vi "_Obtain JKISMQ.vi"(8 "Error in":errorcluster caption="Error in (no error)", 9 "create if not found? (T)":bool=TRUE, 11 "Name(\"\" to use uuid) in":string) -> (0 "Error out":errorcluster, 3 "JKISMQ":T1, 4 "Name":string)   [LabVIEW 2014, in "JKI-State-Machine-Plus.lvlib"]
uses:
  JKI-State-Machine-Plus.lvlib
  _JKISMQ.ctl
  Typedef/_Cross JKI StateMachine State Data.ctl
  Typedef/_JKISM_MSG_TYPE.ctl
  Typedef/_Cross JKI StateMachine State Response.ctl
  Typedef/_JKISM_MODE.ctl
  _JKISMQFGVOPER.ctl
  FGV-BroadcastRegistry/global-JKISMQFGVChangeTStamp.vi
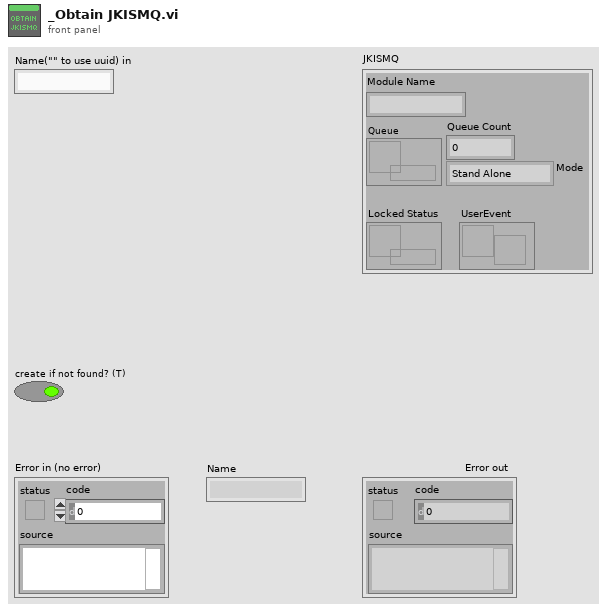
[diagram p1: front panel]
types:
  T1 = typedef "JKI-State-Machine-Plus.lvlib/_JKISMQ.ctl" = cluster{"Module Name":string, "Queue":refnum<queue>, "Locked Status":refnum<data-value>, "Mode":T2, "UserEvent":refnum<user-event>, "Queue Count":i32}
  T2 = typedef "JKI-State-Machine-Plus.lvlib/_JKISM_MODE.ctl" = enum16{"Stand Alone", "JKISM", "Dispatch Worker"}
  T3 = typedef "JKI-State-Machine-Plus.lvlib/_JKISMQFGVOPER.ctl" = enum16{"Get By Name", "List", "Check If Name Exists", "Release", "Module Status"}
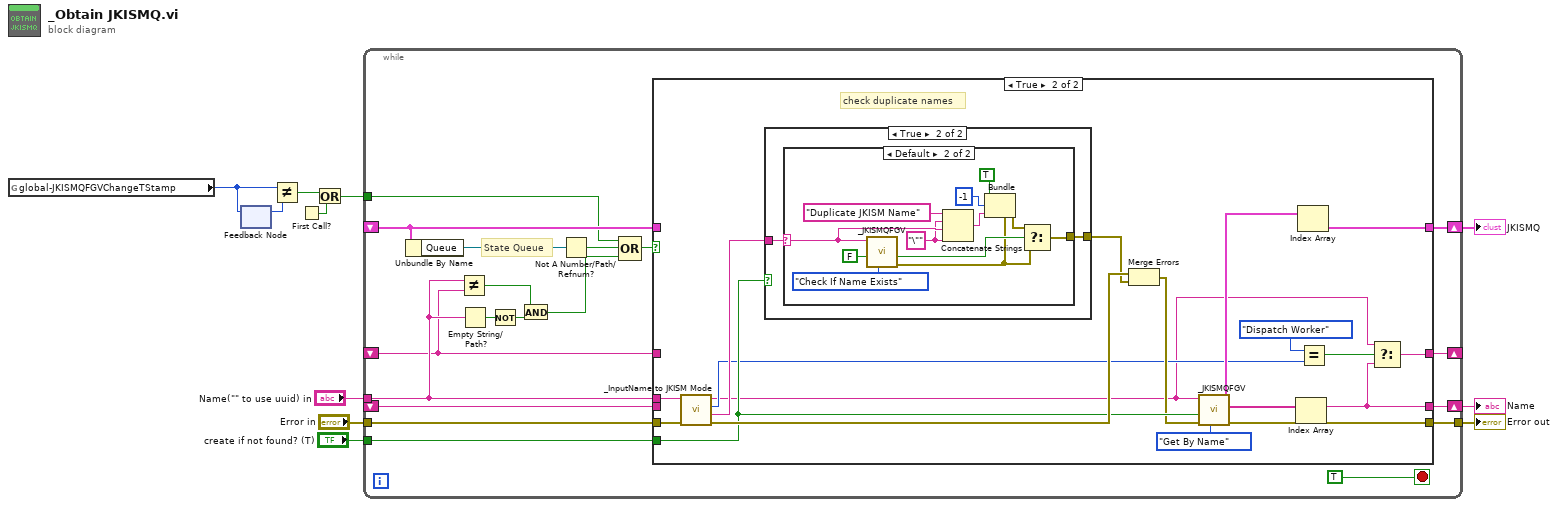
[diagram p0: block diagram]
diagram:
  n1 = global read "global-JKISMQFGVChangeTStamp.vi" "global-JKISMQFGVChangeTStamp"() -> (w2:u32)
  n2 = feedback #1() -> (w3:u32)  [unwired: 1 in]
  n3 = feedback-in #1(w2) -> ()
  n4 = Not Equal?(x=w2, y=w3) -> (x != y?=w5:bool)
  n5 = First Call?() -> (First Call?: T/F=w4:bool)
  n6 = Or(x=w5, y=w4) -> (x .or. y?=w1:bool)
  n7 = while {
    shift-right: [w28] -> w11
    shift-left: _ -> [w23]
    shift-right: [w27] -> w6
    shift-left: _ -> [w19]
    tunnel: "create if not found? (T)" -> [w26]
    tunnel: "Error in" -> [w25]
    tunnel: [w24] -> w8
    tunnel: "Name(\"\" to use uuid) in" -> [w20]
    shift-right: [w14] -> _
    shift-left: _ -> [w13]
    tunnel: w1 -> [w12]
    stop <- TRUE stop-if-true
    # "State Queue"
    n8 = Unbundle By Name(w19) -> ("Queue"=w18:refnum<queue>)
    n9 = Not Equal?(x=w20, y=w13) -> (x != y?=w17:bool)
    n10 = Empty String/Path?(string/path=w20) -> (empty?=w16:bool)
    n11 = Not(x=w16) -> (.not. x?=w15:bool)
    n12 = And(x=w17, y=w15) -> (x .and. y?=w21:bool)
    n13 = Not A Number/Path/Refnum?(number/path/refnum=w18) -> (NaN/Path/Refnum?=w29:bool)
    n14 = Compound Arithmetic op=OR(w12, w29, w21) -> (w22:bool)
    n15 = case shown="True" w22 {
      tunnel: w23 -> [w34 _]
      tunnel: [w34 w36] -> w28
      tunnel: [w33 w43] -> w27
      tunnel: w19 -> [w33 _]
      tunnel: w26 -> [_ w46]
      tunnel: w25 -> [w32 w48]
      tunnel: [w32 w47] -> w24
      tunnel: w20 -> [_ w42]
      tunnel: [w31 w35] -> w14
      tunnel: w13 -> [w31 _]
      frame False {
      }
      frame True {
        # "check duplicate names"
        n16 = call "_InputName to JKISM Mode.vi"("String"=w42) -> ("QName"=w41:string, "JKISM Mode"=w40:T2, "String(dup)"=w37:string)  [unwired: 8 in]
        n17 = case shown="True" w46 {
          tunnel: w41 -> [_ w52]
          tunnel: [_ w53] -> w44
          frame False {
          }
          frame True {
            n18 = case shown="Default" w52 {
              selector: w52 -> [_ w56]
              tunnel: [_ w62] -> w53
              frame "", "PostMessageAPI", "SendMessageAPI" {
              }
              frame Default {
                w55 = "\"" ("string")
                n19 = call "_JKISMQFGV.vi"(6:_JKISMQFGVOPER."Check If Name Exists", "create if not found? (T)"=FALSE, "Name(\"\" to use uuid) in"=w56) -> ("Error out"=w54:errorcluster, "Boolean"=w63:bool)  [unwired: 5 in, 2 out]
                n20 = Concatenate Strings("Duplicate JKISM Name" ("String to Prepend to source (\"\")"), w55, w56, w55) -> (w57:string)
                n21 = Bundle(cluster=w54, "status"=TRUE, "code"=-1, "source"=w57) -> (w61:errorcluster)
                n22 = Select(t=w61, s=w63, f=w54) -> (s? t:f=w62:errorcluster)
              }
            }
          }
        }
        n23 = Merge Errors(w48, w44) -> (w45:errorcluster)
        n24 = call "_JKISMQFGV.vi"(6:_JKISMQFGVOPER."Get By Name", "Error in"=w45, "create if not found? (T)"=w46, "Name(\"\" to use uuid) in"=w37) -> ("Error out"=w47:errorcluster, "Name"=w49:string[], "Array"=w51:T1[])  [unwired: 4 in, 1 out]
        n25 = Index Array(array=w49) -> (element=w36:string)  [unwired: 1 in]
        n26 = Index Array(array=w51) -> (element=w43:T1)  [unwired: 1 in]
        n27 = Equal?(x=_JKISM_MODE."Dispatch Worker", y=w40) -> (x = y?=w38:bool)
        n28 = Select(t=w37, s=w38, f=w36) -> (s? t:f=w35:string)
      }
    }
  }
  "Error out" <- w8
  "JKISMQ" <- w6
  "Name" <- w11
